vi "Replace Log Level Specifier.vi"(11 "format string":string) -> (3 "resulting string":string)   [LabVIEW 2018, in "Logging.lvlib" / "Format String.lvclass"]
uses:
  Format String.lvclass
  <vilib>/regexp/Match Regular Expression.xnode
panel:
  # "Connector Pane"
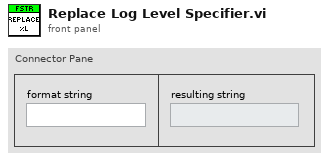
[diagram p1: front panel]
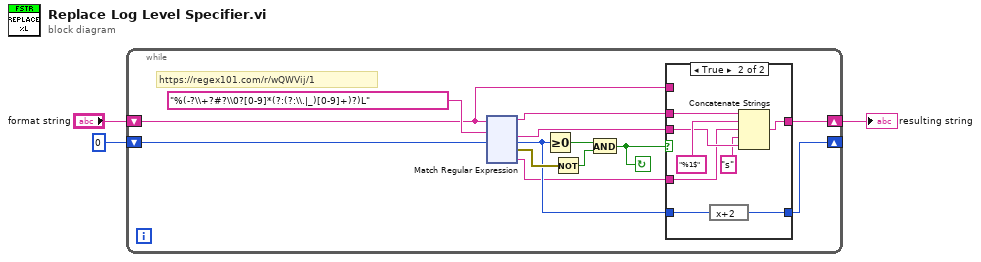
[diagram p0: block diagram]
diagram:
  n1 = while {
    shift-right: [w9] -> w2
    shift-left: "format string" -> [w10]
    shift-right: [w5] -> _
    shift-left: 0 ("offset (0)") -> [w7]
    stop <- w8 continue-if-true
    # "https://regex101.com/r/wQWVij/1"
    n2 = xnode "Match Regular Expression"("input string"=w10, "regular expression"="%(-?\\+?#?\\0?[0-9]*(?:(?:\\.|_)[0-9]+)?)L", "offset (0)"=w7) -> ("before match"=w12:string, "after match"=w11:string, "offset past match"=w6:i32, "error out"=w14:errorcluster, "submatch 1"=w4:string)  [unwired: 3 in, 1 out]
    n3 = Greater Or Equal To 0?(x=w6) -> (x >= 0?=w15:bool)
    n4 = Not(x=w14) -> (.not. x?=w13:bool)
    n5 = And(x=w15, y=w13) -> (x .and. y?=w8:bool)
    n6 = case shown="True" w8 {
      tunnel: w12 -> [_ w145]
      tunnel: w11 -> [_ w143]
      tunnel: [w137 w142] -> w9
      tunnel: w10 -> [w137 _]
      tunnel: w6 -> [w136 w141]
      tunnel: [w136 w140] -> w5
      tunnel: w4 -> [_ w138]
      frame False {
      }
      frame True {
        n7 = expression code="x+2"(w141) -> (w140:i32)
        n8 = Concatenate Strings(w145, "%1$" ("string"), w138, "s" ("string"), w143) -> (w142:string)
      }
    }
  }
  "resulting string" <- w2
